vi "DataRefNew-禁用.vi"(8 "error in (no error)":errorcluster caption="错误输入（无错误）", 11 "MainPage 输入":refnum<class "MainPage.lvclass">) -> (0 "error out":errorcluster caption="错误输出", 2 "数据记录引用":refnum<data-value>, 3 "MainPage 输出":refnum<class "MainPage.lvclass">)   [LabVIEW 2019, in "MainPage.lvlib" / "MainPage.lvclass"]
uses:
  MainPage.lvclass
panel:
  in  "通讯接口记录":T1
  # "弃用，会导致闪退"
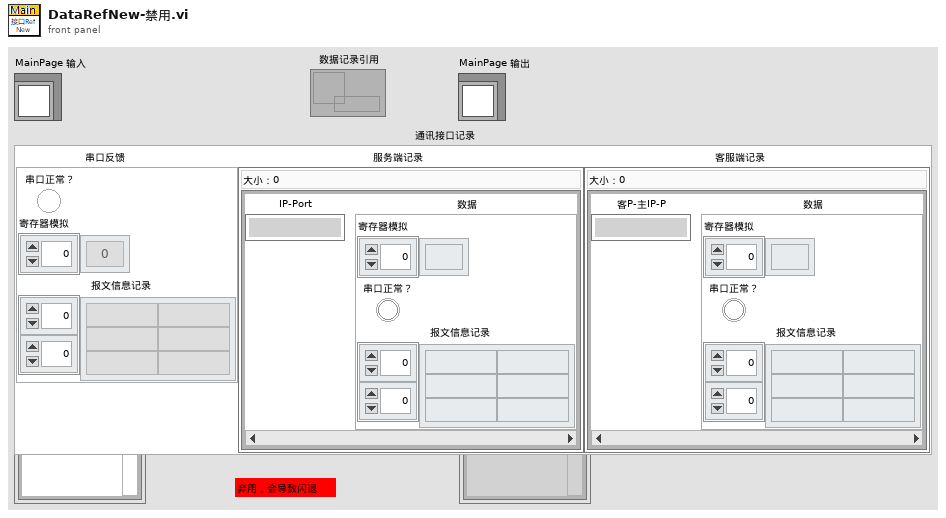
[diagram p1: front panel]
types:
  T1 = typedef "MainPage.lvlib/MainPage.lvclass/DataRef_通讯接口数据记录-弃用.ctl" = cluster{"串口反馈":cluster{"串口正常？":bool, "寄存器模拟":u16[], "报文信息记录":string[][]}, "服务端记录":map{string, cluster{"寄存器模拟":u16[], "串口正常？":bool, "报文信息记录":string[][]}}, "客服端记录":map{string, cluster{"寄存器模拟":u16[], "串口正常？":bool, "报文信息记录":string[][]}}}
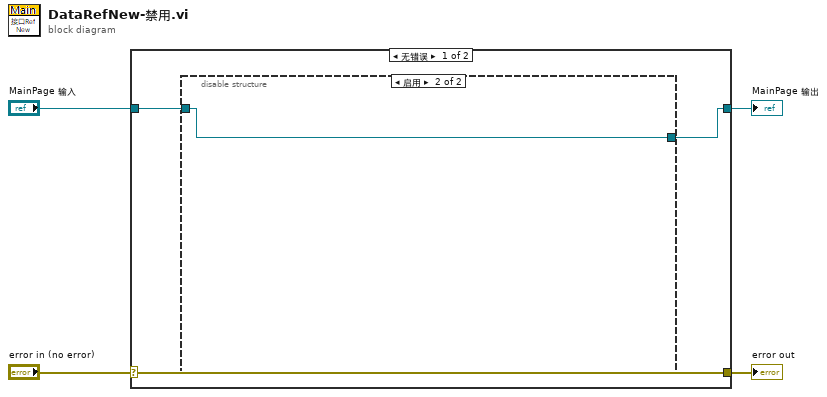
[diagram p0: block diagram]
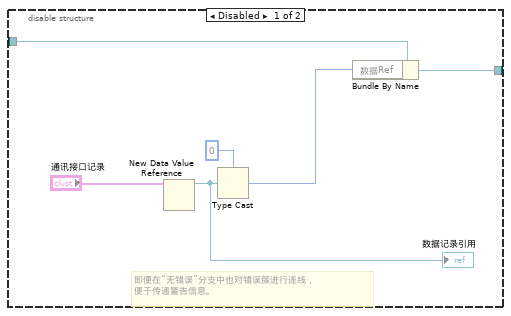
[diagram p2: hidden frame]
diagram:
  n1 = case shown="无错误" "error in (no error)" {
    selector: "error in (no error)" -> [w7 w16]
    tunnel: [w7 w16] -> w3
    tunnel: [w5 w15] -> w1
    tunnel: "MainPage 输入" -> [w6 w15]
    frame No Error {
      n2 = disable-structure shown="启用" {
        disable-tunnel: w6 -> [w11 w14]
        disable-tunnel: [w8 w14] -> w5
        frame Disabled {
          # "即便在“无错误”分支中也对错误簇进行连线，\n便于传递警告信息。"
          n3 = New Data Value Reference(data value="通讯接口记录") -> (data value reference=w9:refnum<data-value>)  [unwired: 1 in, 1 out]
          "数据记录引用" <- w9
          n4 = Type Cast(type=u32 0 ("DataRef"), x=w9) -> (*(type *) &x=w10:u32)
          n5 = Bundle By Name(cluster=w11, "数据Ref"=w10) -> (w8:refnum<class "MainPage.lvclass">)
        }
        frame Enabled {
        }
      }
    }
    frame Error {
    }
  }
  "error out" <- w3
  "MainPage 输出" <- w1
